vi "Determine Cluster Size.vi"(8 "error in":errorcluster, 11 "Variant":variant) -> (0 "error out":errorcluster, 1 "Title":string, 2 "Offsets":i32[](array[numeric]), 3 "Total Size":i32, 4 "SubChannelTitle":string[](array[string]), 5 "DefaultValues":dbl[](array[numeric]), 6 "DataType":string[](array[string]))   [LabVIEW 2023, in "Utilities.lvlib"]
uses:
  Utilities.lvlib
  <vilib>/Utility/Data Type/NI_Data Type.lvlib
  <vilib>/JDP Science/JDP Science Common Utilities/JDP Utility.lvlib
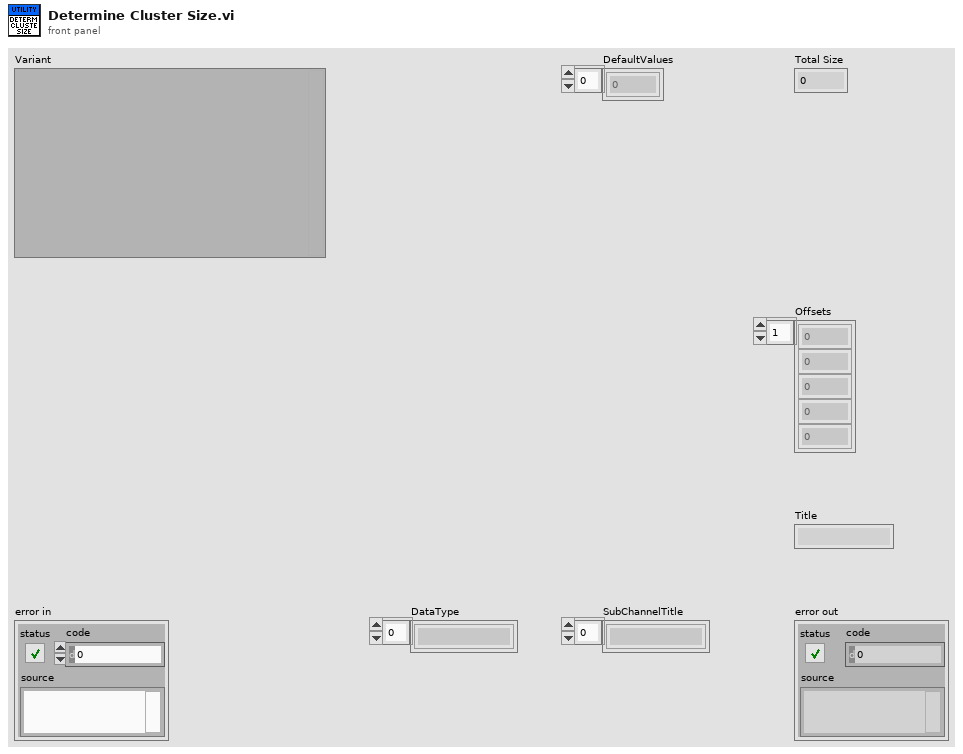
[diagram p1: front panel]
types:
  T1 = typedef "NI_Data Type.lvlib/Data Type.ctl" = enum8{"Invalid Type", "Void", "I8", "I16", "I32", "I64", "U8", "U16", "U32", "U64", "Single Float", "Double Float", "Extended Float", "Single Complex", "Double Complex", "Extended Complex", "Enum U8", "Enum U16", "Enum U32", "Enum U64", "Single Float With Unit", "Double Float With Unit", "Extended Float With Unit", "Single Complex with Unit", "Double Complex with Unit", "Extended Complex with Unit", "Boolean", "String", "Path", "Picture", "Tag", "Array", "Cluster", "Variant", "LV Variant", "Waveform", "Timestamp", "Digital Waveform", "Digital Data", "ExpressData", "Refnum", "External Data", "VI", "Poly VI", "LabVIEW Class Instance", "Fixed Point", "Set Collection", "Map Collection"}
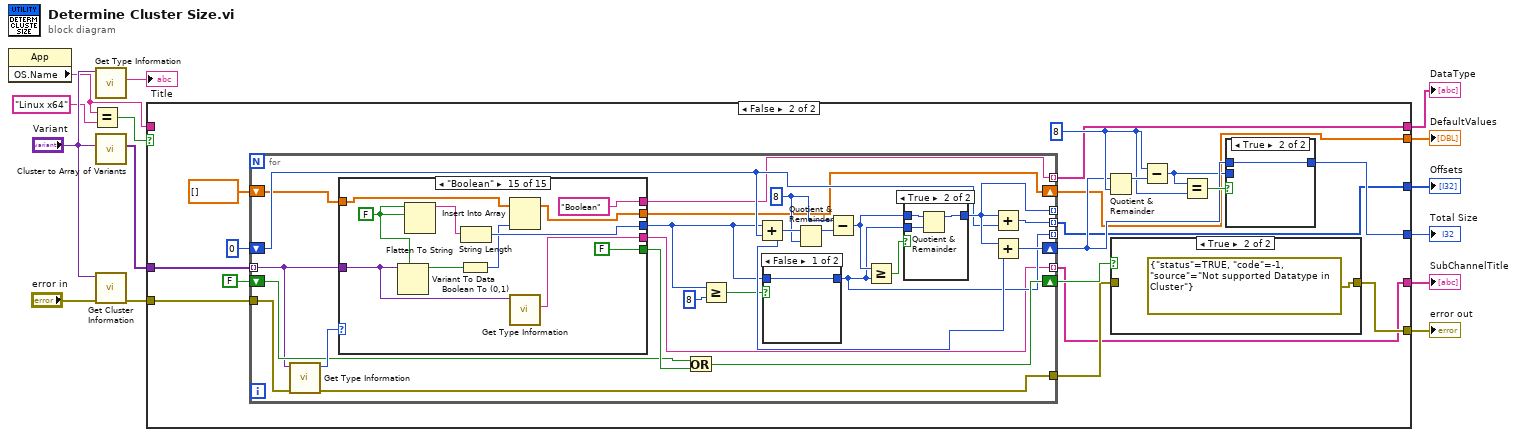
[diagram p0: block diagram]
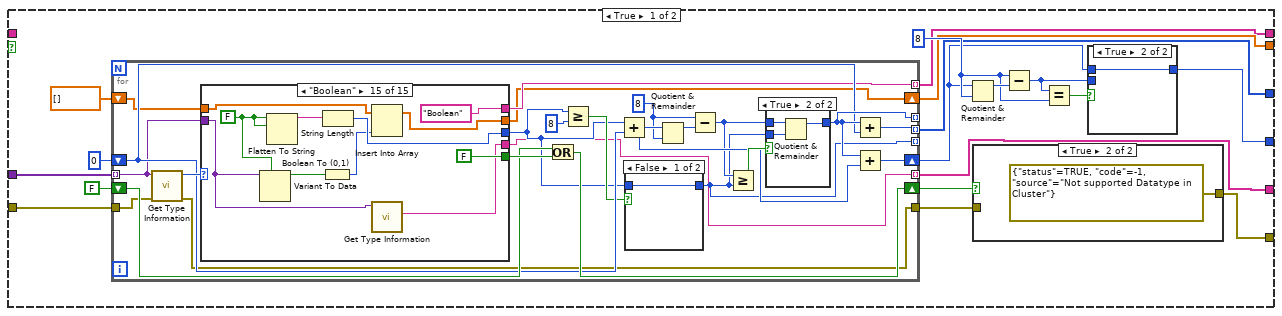
[diagram p2: hidden frame]
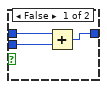
[diagram p4: hidden frame]
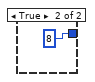
[diagram p5: hidden frame]
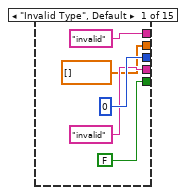
[diagram p7: hidden frame]
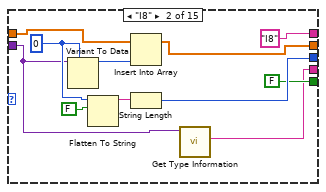
[diagram p8: hidden frame]
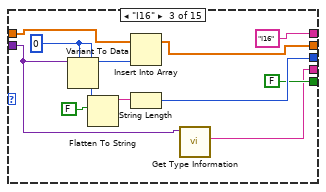
[diagram p9: hidden frame]
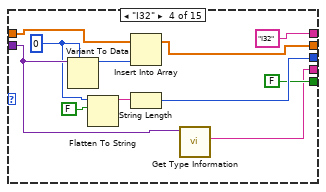
[diagram p10: hidden frame]
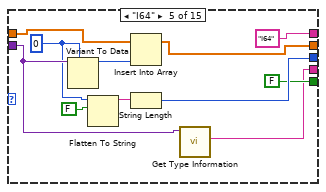
[diagram p11: hidden frame]
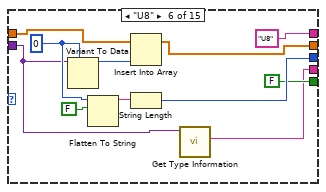
[diagram p12: hidden frame]
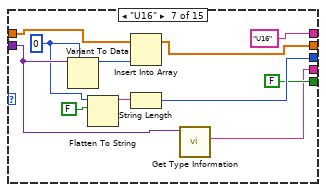
[diagram p13: hidden frame]
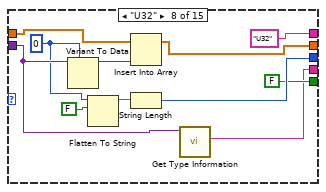
[diagram p14: hidden frame]
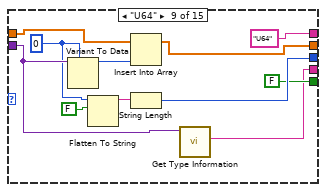
[diagram p15: hidden frame]
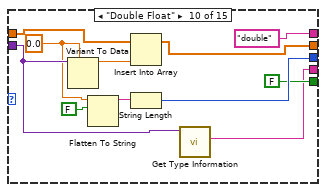
[diagram p16: hidden frame]
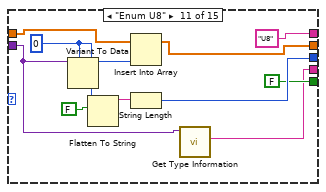
[diagram p17: hidden frame]
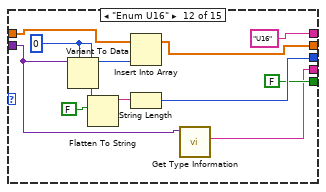
[diagram p18: hidden frame]
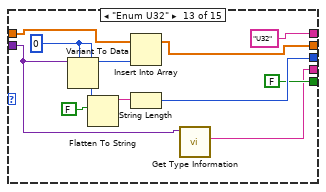
[diagram p19: hidden frame]
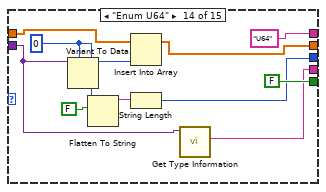
[diagram p20: hidden frame]
diagram:
  n1 = property class="App"() -> ("OS.Name"=w8:string)  [unwired: 2 in, 2 out]
  n2 = Equal?(x=w8, y="Linux x64") -> (x = y?=w7:bool)
  n3 = call <vilib>:"Get Type Information.vi"("variant"="Variant") -> ("name"=→"Title":string)  [unwired: 6 in, 4 out]
  n4 = call <vilib>:"Cluster to Array of Variants.vi"("Cluster"="Variant") -> ("Array of Cluster Elements"=w14:variant[])  [unwired: 10 in]
  n5 = call <vilib>:"Get Cluster Information.vi"("error in (no error)"="error in", "variant"="Variant") -> ("error out"=w12:errorcluster)  [unwired: 8 in, 1 out]
  n6 = case shown="False" w7 {
    tunnel: w14 -> [w24 w237]
    tunnel: [w23 w236] -> w6
    tunnel: w12 -> [w22 w235]
    tunnel: w8 -> [_ _]
    tunnel: [w19 w232] -> w5
    tunnel: [w18 w231] -> w4
    tunnel: [w17 w230] -> w3
    tunnel: [w16 w229] -> w2
    tunnel: [w15 w228] -> w1
    frame True {
      w28 = 8 ("y")
      n7 = for {
        tunnel: [w44] -> _ mode=indexing
        shift-right: [w61] -> w27
        shift-left: 0 -> [w51]
        tunnel: [w50] -> w15 mode=indexing
        tunnel: [w52] -> _ mode=indexing
        shift-right: [w59] -> w25
        shift-left: FALSE -> [w58]
        tunnel: w24 -> [w49] mode=indexing
        tunnel: w22 -> [w48]
        tunnel: [w47] -> w21
        tunnel: [w42] -> w16 mode=indexing
        tunnel: [w41] -> w18 mode=indexing
        shift-right: [w40] -> w19
        shift-left: dbl[] [] -> [w39]
        w54 = 8 ("y")
        n8 = call <vilib>:"Get Type Information.vi"("error in (no error)"=w48, "variant"=w49) -> ("error out"=w47:errorcluster, "type"=w62:T1)  [unwired: 5 in, 3 out]
        n9 = case shown="\"Boolean\"" w62 {
          tunnel: [FALSE FALSE FALSE FALSE FALSE FALSE FALSE FALSE FALSE FALSE FALSE FALSE FALSE FALSE FALSE] -> w60
          tunnel: [0 w82 w93 w104 w115 w126 w137 w148 w159 w170 w181 w192 w203 w213 w225] -> w43
          tunnel: w49 -> [_ w76 w86 w99 w110 w120 w131 w142 w154 w165 w173 w184 w195 w206 w222]
          tunnel: ["invalid" ("name") w80 w90 w101 w112 w124 w134 w145 w156 w168 w178 w189 w200 w211 w223] -> w41
          tunnel: ["invalid" "I8" "I16" "I32" "I64" "U8" "U16" "U32" "U64" "double" "U8" "U16" "U32" "U64" "Boolean"] -> w42
          tunnel: [dbl[] [] w74 w85 w97 w107 w118 w129 w140 w152 w163 w176 w187 w197 w208 w217] -> w40
          tunnel: w39 -> [_ w75 w88 w96 w108 w119 w132 w143 w151 w162 w175 w186 w198 w209 w220]
          frame "Invalid Type", Default {
          }
          frame "I8" {
            w77 = i8 0
            n10 = Variant To Data(type=w77, Variant=w76) -> (data=w78:i8)  [unwired: 1 in, 1 out]
            n11 = Flatten To String(anything=w77, prepend array or string size? (T)=FALSE) -> (data string=w83:string)  [unwired: 2 in, 2 out]
            n12 = Insert Into Array(array=w75, new element=w78) -> (w74:dbl[])  [unwired: 1 in]
            n13 = String Length(string=w83) -> (length=w82:i32)
            n14 = call <vilib>:"Get Type Information.vi"("variant"=w76) -> ("name"=w80:string)  [unwired: 6 in, 4 out]
          }
          frame "I16" {
            w87 = i16 0
            n15 = Variant To Data(type=w87, Variant=w86) -> (data=w89:i16)  [unwired: 1 in, 1 out]
            n16 = Flatten To String(anything=w87, prepend array or string size? (T)=FALSE) -> (data string=w94:string)  [unwired: 2 in, 2 out]
            n17 = Insert Into Array(array=w88, new element=w89) -> (w85:dbl[])  [unwired: 1 in]
            n18 = String Length(string=w94) -> (length=w93:i32)
            n19 = call <vilib>:"Get Type Information.vi"("variant"=w86) -> ("name"=w90:string)  [unwired: 6 in, 4 out]
          }
          frame "I32" {
            w98 = 0
            n20 = Variant To Data(type=w98, Variant=w99) -> (data=w100:i32)  [unwired: 1 in, 1 out]
            n21 = Flatten To String(anything=w98, prepend array or string size? (T)=FALSE) -> (data string=w105:string)  [unwired: 2 in, 2 out]
            n22 = Insert Into Array(array=w96, new element=w100) -> (w97:dbl[])  [unwired: 1 in]
            n23 = String Length(string=w105) -> (length=w104:i32)
            n24 = call <vilib>:"Get Type Information.vi"("variant"=w99) -> ("name"=w101:string)  [unwired: 6 in, 4 out]
          }
          frame "I64" {
            w109 = i64 0
            n25 = Variant To Data(type=w109, Variant=w110) -> (data=w111:i64)  [unwired: 1 in, 1 out]
            n26 = Flatten To String(anything=w109, prepend array or string size? (T)=FALSE) -> (data string=w116:string)  [unwired: 2 in, 2 out]
            n27 = Insert Into Array(array=w108, new element=w111) -> (w107:dbl[])  [unwired: 1 in]
            n28 = String Length(string=w116) -> (length=w115:i32)
            n29 = call <vilib>:"Get Type Information.vi"("variant"=w110) -> ("name"=w112:string)  [unwired: 6 in, 4 out]
          }
          frame "U8" {
            w121 = u8 0
            n30 = Variant To Data(type=w121, Variant=w120) -> (data=w122:u8)  [unwired: 1 in, 1 out]
            n31 = Flatten To String(anything=w121, prepend array or string size? (T)=FALSE) -> (data string=w127:string)  [unwired: 2 in, 2 out]
            n32 = Insert Into Array(array=w119, new element=w122) -> (w118:dbl[])  [unwired: 1 in]
            n33 = String Length(string=w127) -> (length=w126:i32)
            n34 = call <vilib>:"Get Type Information.vi"("variant"=w120) -> ("name"=w124:string)  [unwired: 6 in, 4 out]
          }
          frame "U16" {
            w130 = u16 0
            n35 = Variant To Data(type=w130, Variant=w131) -> (data=w133:u16)  [unwired: 1 in, 1 out]
            n36 = Flatten To String(anything=w130, prepend array or string size? (T)=FALSE) -> (data string=w138:string)  [unwired: 2 in, 2 out]
            n37 = Insert Into Array(array=w132, new element=w133) -> (w129:dbl[])  [unwired: 1 in]
            n38 = String Length(string=w138) -> (length=w137:i32)
            n39 = call <vilib>:"Get Type Information.vi"("variant"=w131) -> ("name"=w134:string)  [unwired: 6 in, 4 out]
          }
          frame "U32" {
            w141 = u32 0
            n40 = Variant To Data(type=w141, Variant=w142) -> (data=w144:u32)  [unwired: 1 in, 1 out]
            n41 = Flatten To String(anything=w141, prepend array or string size? (T)=FALSE) -> (data string=w149:string)  [unwired: 2 in, 2 out]
            n42 = Insert Into Array(array=w143, new element=w144) -> (w140:dbl[])  [unwired: 1 in]
            n43 = String Length(string=w149) -> (length=w148:i32)
            n44 = call <vilib>:"Get Type Information.vi"("variant"=w142) -> ("name"=w145:string)  [unwired: 6 in, 4 out]
          }
          frame "U64" {
            w153 = u64 0
            n45 = Variant To Data(type=w153, Variant=w154) -> (data=w155:u64)  [unwired: 1 in, 1 out]
            n46 = Flatten To String(anything=w153, prepend array or string size? (T)=FALSE) -> (data string=w160:string)  [unwired: 2 in, 2 out]
            n47 = Insert Into Array(array=w151, new element=w155) -> (w152:dbl[])  [unwired: 1 in]
            n48 = String Length(string=w160) -> (length=w159:i32)
            n49 = call <vilib>:"Get Type Information.vi"("variant"=w154) -> ("name"=w156:string)  [unwired: 6 in, 4 out]
          }
          frame "Double Float" {
            w164 = 0.0
            n50 = Variant To Data(type=w164, Variant=w165) -> (data=w166:dbl)  [unwired: 1 in, 1 out]
            n51 = Flatten To String(anything=w164, prepend array or string size? (T)=FALSE) -> (data string=w171:string)  [unwired: 2 in, 2 out]
            n52 = Insert Into Array(array=w162, new element=w166) -> (w163:dbl[])  [unwired: 1 in]
            n53 = String Length(string=w171) -> (length=w170:i32)
            n54 = call <vilib>:"Get Type Information.vi"("variant"=w165) -> ("name"=w168:string)  [unwired: 6 in, 4 out]
          }
          frame "Enum U8" {
            w174 = u8 0
            n55 = Variant To Data(type=w174, Variant=w173) -> (data=w177:u8)  [unwired: 1 in, 1 out]
            n56 = Flatten To String(anything=w174, prepend array or string size? (T)=FALSE) -> (data string=w182:string)  [unwired: 2 in, 2 out]
            n57 = Insert Into Array(array=w175, new element=w177) -> (w176:dbl[])  [unwired: 1 in]
            n58 = String Length(string=w182) -> (length=w181:i32)
            n59 = call <vilib>:"Get Type Information.vi"("variant"=w173) -> ("name"=w178:string)  [unwired: 6 in, 4 out]
          }
          frame "Enum U16" {
            w185 = u16 0
            n60 = Variant To Data(type=w185, Variant=w184) -> (data=w188:u16)  [unwired: 1 in, 1 out]
            n61 = Flatten To String(anything=w185, prepend array or string size? (T)=FALSE) -> (data string=w193:string)  [unwired: 2 in, 2 out]
            n62 = Insert Into Array(array=w186, new element=w188) -> (w187:dbl[])  [unwired: 1 in]
            n63 = String Length(string=w193) -> (length=w192:i32)
            n64 = call <vilib>:"Get Type Information.vi"("variant"=w184) -> ("name"=w189:string)  [unwired: 6 in, 4 out]
          }
          frame "Enum U32" {
            w196 = u32 0
            n65 = Variant To Data(type=w196, Variant=w195) -> (data=w199:u32)  [unwired: 1 in, 1 out]
            n66 = Flatten To String(anything=w196, prepend array or string size? (T)=FALSE) -> (data string=w204:string)  [unwired: 2 in, 2 out]
            n67 = Insert Into Array(array=w198, new element=w199) -> (w197:dbl[])  [unwired: 1 in]
            n68 = String Length(string=w204) -> (length=w203:i32)
            n69 = call <vilib>:"Get Type Information.vi"("variant"=w195) -> ("name"=w200:string)  [unwired: 6 in, 4 out]
          }
          frame "Enum U64" {
            w207 = u64 0
            n70 = Variant To Data(type=w207, Variant=w206) -> (data=w210:u64)  [unwired: 1 in, 1 out]
            n71 = Flatten To String(anything=w207, prepend array or string size? (T)=FALSE) -> (data string=w215:string)  [unwired: 2 in, 2 out]
            n72 = Insert Into Array(array=w209, new element=w210) -> (w208:dbl[])  [unwired: 1 in]
            n73 = String Length(string=w215) -> (length=w213:i32)
            n74 = call <vilib>:"Get Type Information.vi"("variant"=w206) -> ("name"=w211:string)  [unwired: 6 in, 4 out]
          }
          frame "Boolean" {
            w221 = FALSE ("prepend array or string size? (T)")
            n75 = Variant To Data(type=w221, Variant=w222) -> (data=w218:bool)  [unwired: 1 in, 1 out]
            n76 = Flatten To String(anything=w221, prepend array or string size? (T)=w221) -> (data string=w227:string)  [unwired: 2 in, 2 out]
            n77 = Boolean To (0,1)(Boolean=w218) -> (0, 1=w219:i16)
            n78 = String Length(string=w227) -> (length=w225:i32)
            n79 = Insert Into Array(array=w220, new element=w219) -> (w217:dbl[])  [unwired: 1 in]
            n80 = call <vilib>:"Get Type Information.vi"("variant"=w222) -> ("name"=w223:string)  [unwired: 6 in, 4 out]
          }
        }
        n81 = Or(x=w58, y=w60) -> (x .or. y?=w59:bool)
        n82 = Greater Or Equal?(x=w43, y=8) -> (x >= y?=w45:bool)
        n83 = Add(x=w43, y=w51) -> (x+y=w56:i32)
        n84 = case shown="False" w45 {
          tunnel: [w63 8 ("y")] -> w44
          tunnel: w43 -> [w63 _]
          frame False {
          }
          frame True {
          }
        }
        n85 = Quotient & Remainder(x=w56, y=w54) -> (x-y*floor(x/y)=w55:i32)  [unwired: 1 out]
        n86 = Subtract(x=w54, y=w55) -> (x-y=w53:i32)
        n87 = Greater Or Equal?(x=w53, y=w44) -> (x >= y?=w57:bool)
        n88 = case shown="True" w57 {
          tunnel: [w65 w66] -> w52
          tunnel: w53 -> [w65 w68]
          tunnel: w44 -> [_ w67]
          frame False {
          }
          frame True {
            n89 = Quotient & Remainder(x=w68, y=w67) -> (x-y*floor(x/y)=w66:i32)  [unwired: 1 out]
          }
        }
        n90 = Add(x=w52, y=w51) -> (x+y=w50:i32)
        n91 = Add(x=w52, y=w56) -> (x+y=w61:i32)
      }
      n92 = Quotient & Remainder(x=w27, y=w28) -> (x-y*floor(x/y)=w30:i32)  [unwired: 1 out]
      n93 = case shown="True" w25 {
        tunnel: w21 -> [w33 _]
        tunnel: [w33 errorcluster {"status"=TRUE, "code"=-1, "source"="Not supported Datatype in Cluster"} ("error in")] -> w23
        frame False {
        }
        frame True {
        }
      }
      n94 = Subtract(x=w28, y=w30) -> (x-y=w26:i32)
      n95 = Equal?(x=w26, y=w28) -> (x = y?=w29:bool)
      n96 = case shown="True" w29 {
        tunnel: w27 -> [w37 w38]
        tunnel: [w36 w38] -> w17
        tunnel: w26 -> [w35 _]
        frame False {
          n97 = Add(x=w37, y=w35) -> (x+y=w36:i32)
        }
        frame True {
        }
      }
    }
    frame False {
      w241 = 8 ("y")
      n98 = for {
        tunnel: [w257] -> _ mode=indexing
        shift-right: [w274] -> w240
        shift-left: 0 -> [w264]
        tunnel: [w263] -> w228 mode=indexing
        tunnel: [w265] -> _ mode=indexing
        shift-right: [w272] -> w238
        shift-left: FALSE -> [w271]
        tunnel: w237 -> [w262] mode=indexing
        tunnel: w235 -> [w261]
        tunnel: [w260] -> w234
        tunnel: [w255] -> w229 mode=indexing
        tunnel: [w254] -> w231 mode=indexing
        shift-right: [w253] -> w232
        shift-left: dbl[] [] -> [w252]
        w267 = 8 ("y")
        n99 = call <vilib>:"Get Type Information.vi"("error in (no error)"=w261, "variant"=w262) -> ("error out"=w260:errorcluster, "type"=w275:T1)  [unwired: 5 in, 3 out]
        n100 = case shown="\"Boolean\"" w275 {
          tunnel: [FALSE FALSE FALSE FALSE FALSE FALSE FALSE FALSE FALSE FALSE FALSE FALSE FALSE FALSE FALSE] -> w273
          tunnel: [0 w295 w306 w317 w328 w339 w350 w361 w372 w383 w394 w405 w416 w426 w438] -> w256
          tunnel: w262 -> [_ w289 w299 w312 w323 w333 w344 w355 w367 w378 w386 w397 w408 w419 w435]
          tunnel: ["invalid" ("name") w293 w303 w314 w325 w337 w347 w358 w369 w381 w391 w402 w413 w424 w436] -> w254
          tunnel: ["invalid" "I8" "I16" "I32" "I64" "U8" "U16" "U32" "U64" "double" "U8" "U16" "U32" "U64" "Boolean"] -> w255
          tunnel: [dbl[] [] w287 w298 w310 w320 w331 w342 w353 w365 w376 w389 w400 w410 w421 w430] -> w253
          tunnel: w252 -> [_ w288 w301 w309 w321 w332 w345 w356 w364 w375 w388 w399 w411 w422 w433]
          frame "Invalid Type", Default {
          }
          frame "I8" {
            w290 = i8 0
            n101 = Variant To Data(type=w290, Variant=w289) -> (data=w291:i8)  [unwired: 1 in, 1 out]
            n102 = Flatten To String(anything=w290, prepend array or string size? (T)=FALSE) -> (data string=w296:string)  [unwired: 2 in, 2 out]
            n103 = Insert Into Array(array=w288, new element=w291) -> (w287:dbl[])  [unwired: 1 in]
            n104 = String Length(string=w296) -> (length=w295:i32)
            n105 = call <vilib>:"Get Type Information.vi"("variant"=w289) -> ("name"=w293:string)  [unwired: 6 in, 4 out]
          }
          frame "I16" {
            w300 = i16 0
            n106 = Variant To Data(type=w300, Variant=w299) -> (data=w302:i16)  [unwired: 1 in, 1 out]
            n107 = Flatten To String(anything=w300, prepend array or string size? (T)=FALSE) -> (data string=w307:string)  [unwired: 2 in, 2 out]
            n108 = Insert Into Array(array=w301, new element=w302) -> (w298:dbl[])  [unwired: 1 in]
            n109 = String Length(string=w307) -> (length=w306:i32)
            n110 = call <vilib>:"Get Type Information.vi"("variant"=w299) -> ("name"=w303:string)  [unwired: 6 in, 4 out]
          }
          frame "I32" {
            w311 = 0
            n111 = Variant To Data(type=w311, Variant=w312) -> (data=w313:i32)  [unwired: 1 in, 1 out]
            n112 = Flatten To String(anything=w311, prepend array or string size? (T)=FALSE) -> (data string=w318:string)  [unwired: 2 in, 2 out]
            n113 = Insert Into Array(array=w309, new element=w313) -> (w310:dbl[])  [unwired: 1 in]
            n114 = String Length(string=w318) -> (length=w317:i32)
            n115 = call <vilib>:"Get Type Information.vi"("variant"=w312) -> ("name"=w314:string)  [unwired: 6 in, 4 out]
          }
          frame "I64" {
            w322 = i64 0
            n116 = Variant To Data(type=w322, Variant=w323) -> (data=w324:i64)  [unwired: 1 in, 1 out]
            n117 = Flatten To String(anything=w322, prepend array or string size? (T)=FALSE) -> (data string=w329:string)  [unwired: 2 in, 2 out]
            n118 = Insert Into Array(array=w321, new element=w324) -> (w320:dbl[])  [unwired: 1 in]
            n119 = String Length(string=w329) -> (length=w328:i32)
            n120 = call <vilib>:"Get Type Information.vi"("variant"=w323) -> ("name"=w325:string)  [unwired: 6 in, 4 out]
          }
          frame "U8" {
            w334 = u8 0
            n121 = Variant To Data(type=w334, Variant=w333) -> (data=w335:u8)  [unwired: 1 in, 1 out]
            n122 = Flatten To String(anything=w334, prepend array or string size? (T)=FALSE) -> (data string=w340:string)  [unwired: 2 in, 2 out]
            n123 = Insert Into Array(array=w332, new element=w335) -> (w331:dbl[])  [unwired: 1 in]
            n124 = String Length(string=w340) -> (length=w339:i32)
            n125 = call <vilib>:"Get Type Information.vi"("variant"=w333) -> ("name"=w337:string)  [unwired: 6 in, 4 out]
          }
          frame "U16" {
            w343 = u16 0
            n126 = Variant To Data(type=w343, Variant=w344) -> (data=w346:u16)  [unwired: 1 in, 1 out]
            n127 = Flatten To String(anything=w343, prepend array or string size? (T)=FALSE) -> (data string=w351:string)  [unwired: 2 in, 2 out]
            n128 = Insert Into Array(array=w345, new element=w346) -> (w342:dbl[])  [unwired: 1 in]
            n129 = String Length(string=w351) -> (length=w350:i32)
            n130 = call <vilib>:"Get Type Information.vi"("variant"=w344) -> ("name"=w347:string)  [unwired: 6 in, 4 out]
          }
          frame "U32" {
            w354 = u32 0
            n131 = Variant To Data(type=w354, Variant=w355) -> (data=w357:u32)  [unwired: 1 in, 1 out]
            n132 = Flatten To String(anything=w354, prepend array or string size? (T)=FALSE) -> (data string=w362:string)  [unwired: 2 in, 2 out]
            n133 = Insert Into Array(array=w356, new element=w357) -> (w353:dbl[])  [unwired: 1 in]
            n134 = String Length(string=w362) -> (length=w361:i32)
            n135 = call <vilib>:"Get Type Information.vi"("variant"=w355) -> ("name"=w358:string)  [unwired: 6 in, 4 out]
          }
          frame "U64" {
            w366 = u64 0
            n136 = Variant To Data(type=w366, Variant=w367) -> (data=w368:u64)  [unwired: 1 in, 1 out]
            n137 = Flatten To String(anything=w366, prepend array or string size? (T)=FALSE) -> (data string=w373:string)  [unwired: 2 in, 2 out]
            n138 = Insert Into Array(array=w364, new element=w368) -> (w365:dbl[])  [unwired: 1 in]
            n139 = String Length(string=w373) -> (length=w372:i32)
            n140 = call <vilib>:"Get Type Information.vi"("variant"=w367) -> ("name"=w369:string)  [unwired: 6 in, 4 out]
          }
          frame "Double Float" {
            w377 = 0.0
            n141 = Variant To Data(type=w377, Variant=w378) -> (data=w379:dbl)  [unwired: 1 in, 1 out]
            n142 = Flatten To String(anything=w377, prepend array or string size? (T)=FALSE) -> (data string=w384:string)  [unwired: 2 in, 2 out]
            n143 = Insert Into Array(array=w375, new element=w379) -> (w376:dbl[])  [unwired: 1 in]
            n144 = String Length(string=w384) -> (length=w383:i32)
            n145 = call <vilib>:"Get Type Information.vi"("variant"=w378) -> ("name"=w381:string)  [unwired: 6 in, 4 out]
          }
          frame "Enum U8" {
            w387 = u8 0
            n146 = Variant To Data(type=w387, Variant=w386) -> (data=w390:u8)  [unwired: 1 in, 1 out]
            n147 = Flatten To String(anything=w387, prepend array or string size? (T)=FALSE) -> (data string=w395:string)  [unwired: 2 in, 2 out]
            n148 = Insert Into Array(array=w388, new element=w390) -> (w389:dbl[])  [unwired: 1 in]
            n149 = String Length(string=w395) -> (length=w394:i32)
            n150 = call <vilib>:"Get Type Information.vi"("variant"=w386) -> ("name"=w391:string)  [unwired: 6 in, 4 out]
          }
          frame "Enum U16" {
            w398 = u16 0
            n151 = Variant To Data(type=w398, Variant=w397) -> (data=w401:u16)  [unwired: 1 in, 1 out]
            n152 = Flatten To String(anything=w398, prepend array or string size? (T)=FALSE) -> (data string=w406:string)  [unwired: 2 in, 2 out]
            n153 = Insert Into Array(array=w399, new element=w401) -> (w400:dbl[])  [unwired: 1 in]
            n154 = String Length(string=w406) -> (length=w405:i32)
            n155 = call <vilib>:"Get Type Information.vi"("variant"=w397) -> ("name"=w402:string)  [unwired: 6 in, 4 out]
          }
          frame "Enum U32" {
            w409 = u32 0
            n156 = Variant To Data(type=w409, Variant=w408) -> (data=w412:u32)  [unwired: 1 in, 1 out]
            n157 = Flatten To String(anything=w409, prepend array or string size? (T)=FALSE) -> (data string=w417:string)  [unwired: 2 in, 2 out]
            n158 = Insert Into Array(array=w411, new element=w412) -> (w410:dbl[])  [unwired: 1 in]
            n159 = String Length(string=w417) -> (length=w416:i32)
            n160 = call <vilib>:"Get Type Information.vi"("variant"=w408) -> ("name"=w413:string)  [unwired: 6 in, 4 out]
          }
          frame "Enum U64" {
            w420 = u64 0
            n161 = Variant To Data(type=w420, Variant=w419) -> (data=w423:u64)  [unwired: 1 in, 1 out]
            n162 = Flatten To String(anything=w420, prepend array or string size? (T)=FALSE) -> (data string=w428:string)  [unwired: 2 in, 2 out]
            n163 = Insert Into Array(array=w422, new element=w423) -> (w421:dbl[])  [unwired: 1 in]
            n164 = String Length(string=w428) -> (length=w426:i32)
            n165 = call <vilib>:"Get Type Information.vi"("variant"=w419) -> ("name"=w424:string)  [unwired: 6 in, 4 out]
          }
          frame "Boolean" {
            w434 = FALSE ("prepend array or string size? (T)")
            n166 = Variant To Data(type=w434, Variant=w435) -> (data=w431:bool)  [unwired: 1 in, 1 out]
            n167 = Flatten To String(anything=w434, prepend array or string size? (T)=w434) -> (data string=w440:string)  [unwired: 2 in, 2 out]
            n168 = Boolean To (0,1)(Boolean=w431) -> (0, 1=w432:i16)
            n169 = String Length(string=w440) -> (length=w438:i32)
            n170 = Insert Into Array(array=w433, new element=w432) -> (w430:dbl[])  [unwired: 1 in]
            n171 = call <vilib>:"Get Type Information.vi"("variant"=w435) -> ("name"=w436:string)  [unwired: 6 in, 4 out]
          }
        }
        n172 = Or(x=w271, y=w273) -> (x .or. y?=w272:bool)
        n173 = Greater Or Equal?(x=w256, y=8) -> (x >= y?=w258:bool)
        n174 = Add(x=w256, y=w264) -> (x+y=w269:i32)
        n175 = case shown="False" w258 {
          tunnel: [w276 8 ("y")] -> w257
          tunnel: w256 -> [w276 _]
          frame False {
          }
          frame True {
          }
        }
        n176 = Quotient & Remainder(x=w269, y=w267) -> (x-y*floor(x/y)=w268:i32)  [unwired: 1 out]
        n177 = Subtract(x=w267, y=w268) -> (x-y=w266:i32)
        n178 = Greater Or Equal?(x=w266, y=w257) -> (x >= y?=w270:bool)
        n179 = case shown="True" w270 {
          tunnel: [w278 w279] -> w265
          tunnel: w266 -> [w278 w281]
          tunnel: w257 -> [_ w280]
          frame False {
          }
          frame True {
            n180 = Quotient & Remainder(x=w281, y=w280) -> (x-y*floor(x/y)=w279:i32)  [unwired: 1 out]
          }
        }
        n181 = Add(x=w265, y=w264) -> (x+y=w263:i32)
        n182 = Add(x=w265, y=w269) -> (x+y=w274:i32)
      }
      n183 = Quotient & Remainder(x=w240, y=w241) -> (x-y*floor(x/y)=w243:i32)  [unwired: 1 out]
      n184 = case shown="True" w238 {
        tunnel: w234 -> [w246 _]
        tunnel: [w246 errorcluster {"status"=TRUE, "code"=-1, "source"="Not supported Datatype in Cluster"} ("error in")] -> w236
        frame False {
        }
        frame True {
        }
      }
      n185 = Subtract(x=w241, y=w243) -> (x-y=w239:i32)
      n186 = Equal?(x=w239, y=w241) -> (x = y?=w242:bool)
      n187 = case shown="True" w242 {
        tunnel: w240 -> [w250 w251]
        tunnel: [w249 w251] -> w230
        tunnel: w239 -> [w248 _]
        frame False {
          n188 = Add(x=w250, y=w248) -> (x+y=w249:i32)
        }
        frame True {
        }
      }
    }
  }
  "error out" <- w6
  "SubChannelTitle" <- w4
  "DefaultValues" <- w5
  "Total Size" <- w3
  "DataType" <- w2
  "Offsets" <- w1
